vi "SwitchBoard_switch.vi"(8 "error in":errorcluster, 10 "Channel":i32, 11 "Handle":u32) -> (0 "error out":errorcluster, 3 "Handle":u32)   [LabVIEW 2016]
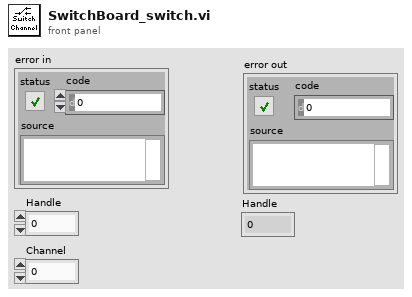
[diagram p1: front panel]
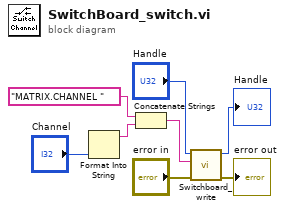
[diagram p0: block diagram]
diagram:
  n1 = Format Into String("Channel") -> (resulting string=w1:string)  [unwired: 3 in, 1 out]
  n2 = Concatenate Strings("MATRIX.CHANNEL " ("string"), w1) -> (w7:string)
  n3 = call "Switchboard_write.vi"("error in"="error in", "Buffer"=w7, "Handle"="Handle") -> ("error out"=→"error out":errorcluster, "Handle"=→"Handle":u32)  [unwired: 6 in, 1 out]
